vi "TickTock.vi"(8 "Error In":errorcluster, 11 "Current Time (In)":timestamp) -> (0 "Error Out":errorcluster, 2 "dt":dbl, 3 "Current Time (Out)":timestamp)   [LabVIEW 2018]
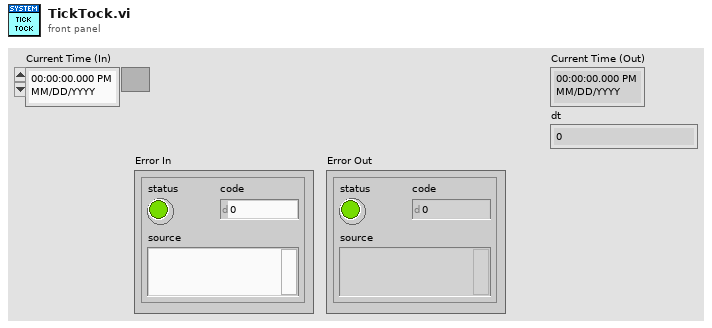
[diagram p1: front panel]
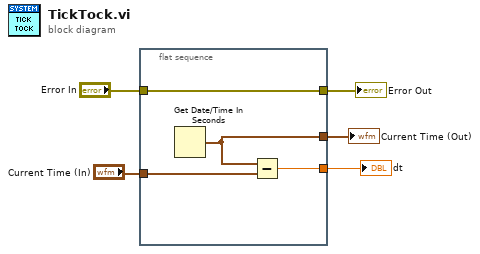
[diagram p0: block diagram]
diagram:
  n1 = flat-sequence {
    tunnel: [w9] -> w5
    tunnel: "Current Time (In)" -> [w8]
    tunnel: [w7] -> w3
    tunnel: [w6] -> w2
    tunnel: "Error In" -> [w6]
    frame #0 {
      n2 = Get Date/Time In Seconds() -> (seconds since 1Jan1904=w9:timestamp)
      n3 = Subtract(x=w9, y=w8) -> (x-y=w7:dbl)
    }
  }
  "Current Time (Out)" <- w5
  "dt" <- w3
  "Error Out" <- w2
